vi "GetMeas.vi"(0 "VISA resource name":refnum<visa-resource-name>) -> (1 "Measure":dbl, 2 "Count":dbl)   [LabVIEW 2014]
panel:
  out "element":string
  out "array":string[](array[string])
  out "read buffer":string
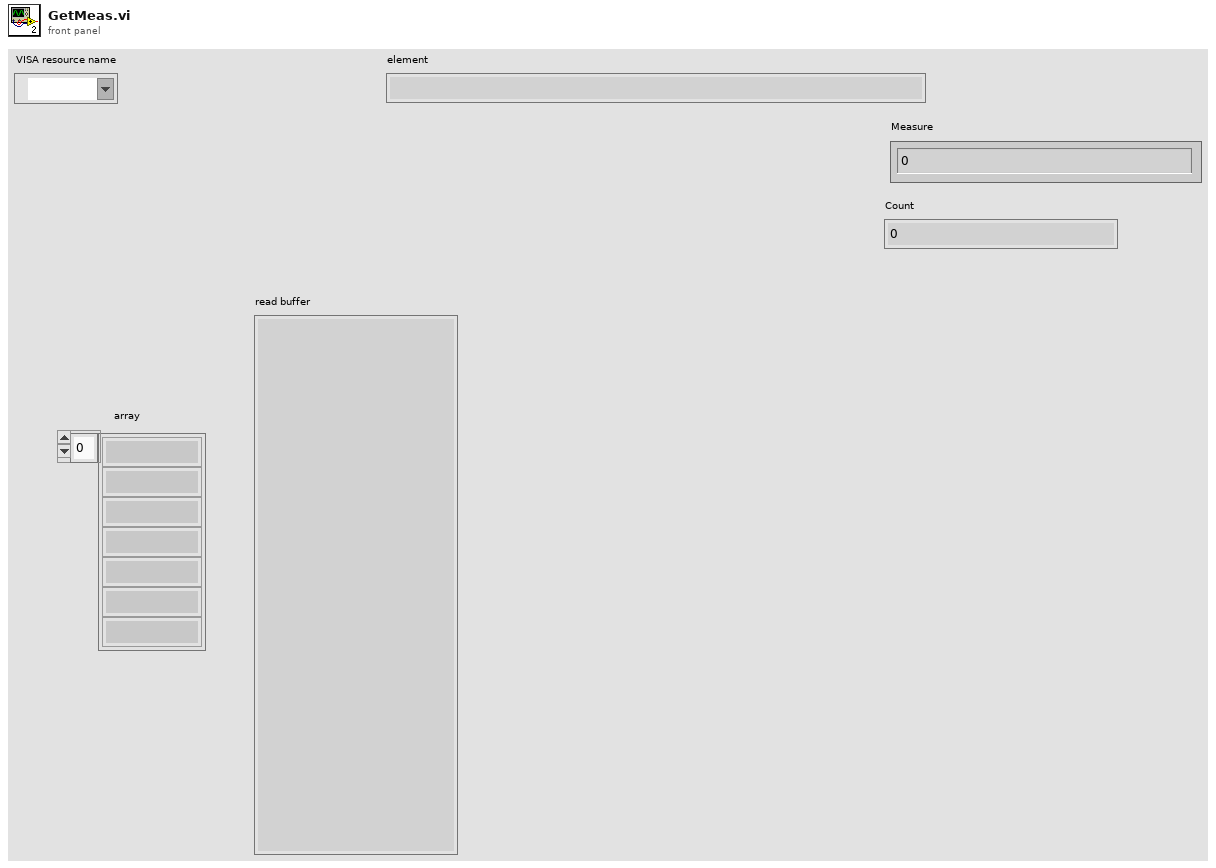
[diagram p1: front panel]
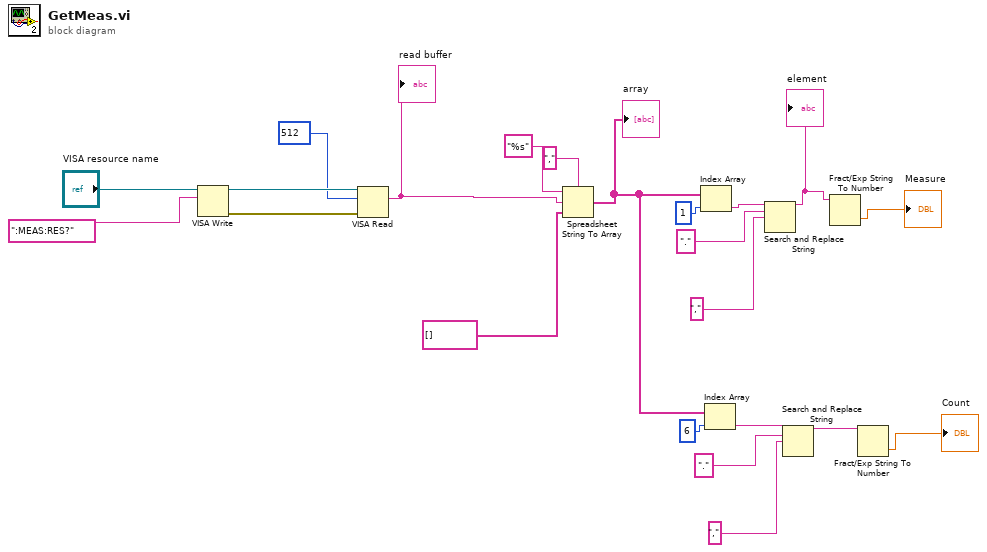
[diagram p0: block diagram]
diagram:
  n1 = VISA Write(VISA resource name="VISA resource name", write buffer=":MEAS:RES?") -> (VISA resource name out=w22:refnum<visa-resource-name>, error out=w21:errorcluster)  [unwired: 1 in, 1 out]
  n2 = VISA Read(VISA resource name=w22, byte count=u32 512, error in (no error)=w21) -> (read buffer=w18:string)  [unwired: 3 out]
  "read buffer" <- w18
  n3 = Spreadsheet String To Array(delimiter (Tab)=",", format string="%s", spreadsheet string=w18, array type (2D Dbl)=string[] []) -> (array=w7:string[])
  "array" <- w7
  n4 = Index Array(array=w7, index=1) -> (element=w12:string)
  n5 = Index Array(array=w7, index=6) -> (element=w6:string)
  n6 = Search and Replace String(input string=w12, search string=".", replace string="," ("replace string (\"\")")) -> (result string=w9:string)  [unwired: 5 in, 3 out]
  "element" <- w9
  n7 = Search and Replace String(input string=w6, search string=".", replace string="," ("replace string (\"\")")) -> (result string=w3:string)  [unwired: 5 in, 3 out]
  n8 = Fract/Exp String To Number(string=w9) -> (number=→"Measure":dbl)  [unwired: 3 in, 1 out]
  n9 = Fract/Exp String To Number(string=w3) -> (number=→"Count":dbl)  [unwired: 3 in, 1 out]
